vi "Conv2D(LabVIEW).vi"() -> ()   [LabVIEW 2020]
uses:
  725156de-cf75-4898-947e-c29841973b14.vi
  dd0536cf-4951-4d31-99bd-6811dd0ed3e3.vi
  <vilib>/Utility/High Resolution Relative Seconds.vi
  <vilib>/Analysis/baseanly.llb/Mean (DBL).vi
  <vilib>/Analysis/2dsp.llb/2D Convolution (DBL).vi
  <vilib>/Utility/file.llb/Write Delimited Spreadsheet (DBL).vi
  <vilib>/Analysis/NI_AALBase.lvlib
  <vilib>/Analysis/NI_AALPro.lvlib
panel:
  out "Results(s)":dbl[][](array[numeric])=[[0.00042240900000251714, 0.0006797469999992245, 0.001307318000003761, 0.0018059579999999188, 0.0029984490000015285, 0.0035659910000003948, 0.005167819000002964], [0.0016064430000005813, 0.002645904999999402, 0.0053270980000024795, 0.007167966000001798, 0.011575462000000697, 0.01364413499999955, 0.01941537100000005], [0.006691304000000855, 0.010726035000002411, 0.020936882000000878, 0.027458231000000523, 0.04479016899999806, 0.05343978200000038, 0.07617650899999717], [0.027480451999999787, 0.042863392000003844, 0.08360431799999787, 0.11047097800000301, 0.17862831899999945, 0.21162874799999826, 0.29438628300000347], [0.11078803599999901, 0.17429765300000327, 0.331365909000001, 0.4447229849999985, 0.7105940409999993, 0.886198787000003, 1.1901550199999975]] format="%.2f"
  in  "algorithm":enum32{"direct", "frequency domain"}(ring)
  in  "Kernel Size":i32[](array[numeric])=[3, 5, 7, 9, 11, 13, 15]
  in  "Image Size":i32[](array[numeric])=[128, 256, 512, 1024, 2048]
  in  "Batch":i32=100
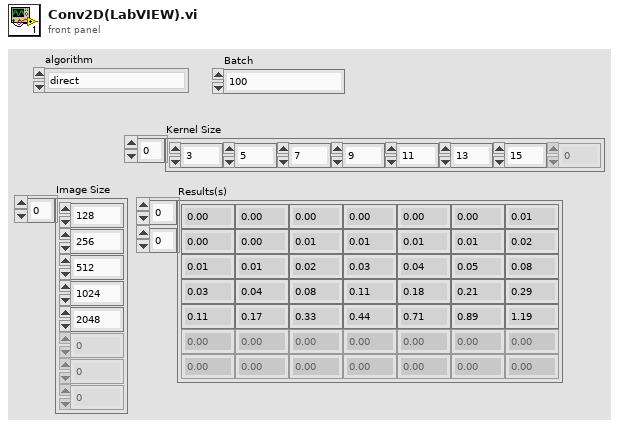
[diagram p1: front panel]
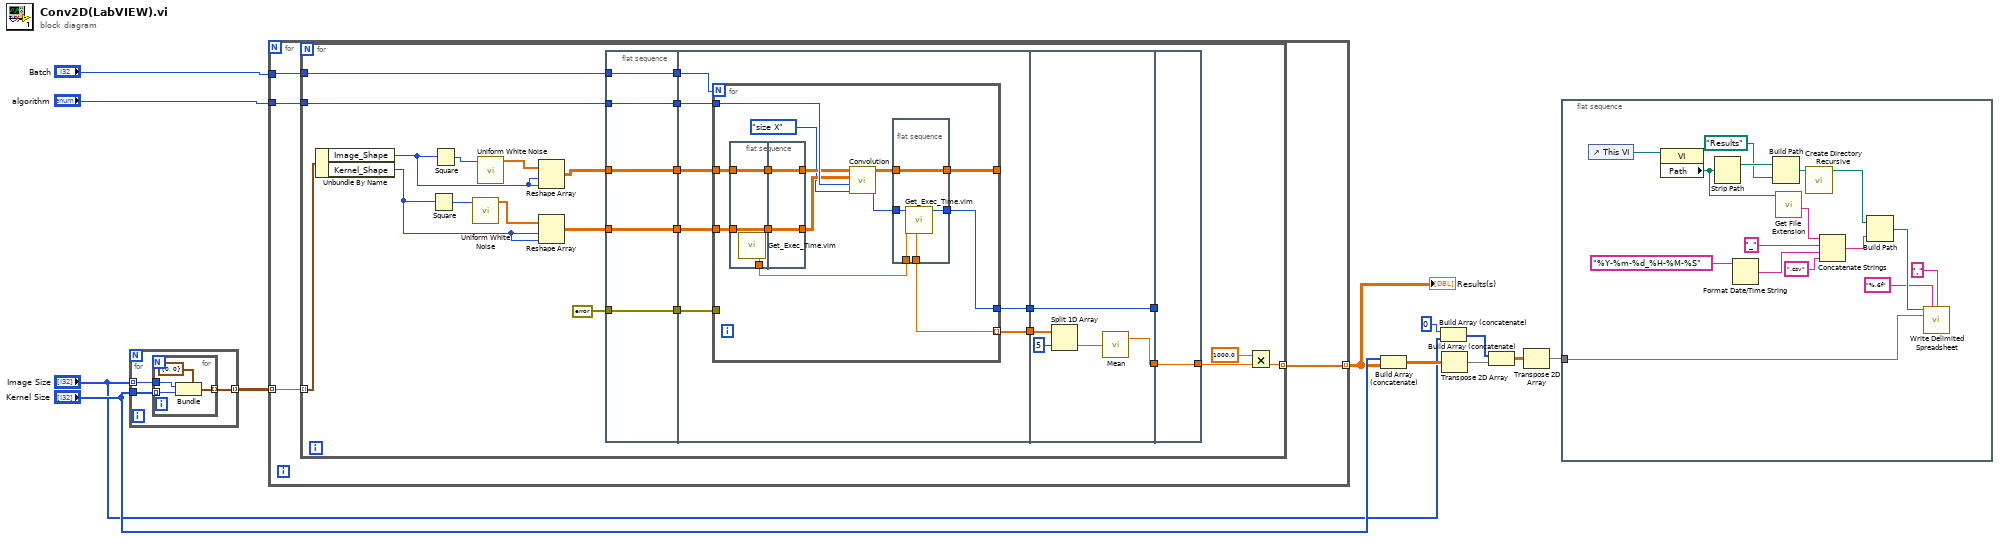
[diagram p0: block diagram]
diagram:
  n1 = for {
    tunnel: "Image Size" -> [w14] mode=indexing
    tunnel: "Kernel Size" -> [w15]
    tunnel: [w13] -> w1 mode=indexing
    n2 = for {
      tunnel: w15 -> [w18] mode=indexing
      tunnel: w14 -> [w19]
      tunnel: [w17] -> w13 mode=indexing
      n3 = Bundle(cluster=cluster{"Image_Shape":i32, "Kernel_Shape":i32} {"Image_Shape"=0, "Kernel_Shape"=0}, "Image_Shape"=w19, "Kernel_Shape"=w18) -> (w17:cluster{"Image_Shape":i32, "Kernel_Shape":i32})
    }
  }
  n4 = for {
    tunnel: w1 -> [w23] mode=indexing
    tunnel: "Batch" -> [w20]
    tunnel: [w22] -> w4 mode=indexing
    tunnel: "algorithm" -> [w21]
    n5 = for {
      tunnel: w23 -> [w47] mode=indexing
      tunnel: [w26] -> w22 mode=indexing
      tunnel: w21 -> [w29]
      tunnel: w20 -> [w28]
      n6 = Unbundle By Name(w47) -> ("Image_Shape"=w38:i32, "Kernel_Shape"=w42:i32)
      n7 = Square(x=w42) -> (x^2=w39:i32)
      n8 = Square(x=w38) -> (x^2=w27:i32)
      n9 = call <vilib>:"Uniform White Noise.vi"("samples"=w39) -> ("uniform white noise"=w40:dbl[])  [unwired: 9 in, 1 out]
      n10 = call <vilib>:"Uniform White Noise.vi"("samples"=w27) -> ("uniform white noise"=w41:dbl[])  [unwired: 9 in, 1 out]
      n11 = Reshape Array(w41, w38, w38) -> (w33:dbl[][])
      n12 = Reshape Array(w40, w42, w42) -> (w43:dbl[][])
      n13 = flat-sequence {
        tunnel: w29 -> [w50]
        tunnel: errorcluster {"status"=FALSE, "code"=0, "source"=""} ("error out") -> [w49]
        tunnel: w43 -> [w51]
        tunnel: w33 -> [w52]
        tunnel: [w52] -> w37
        tunnel: [w51] -> w36
        tunnel: [w49] -> w35
        tunnel: [w50] -> w34
        tunnel: [w48] -> w32
        tunnel: w28 -> [w48]
        tunnel: [w56] -> w46
        tunnel: w37 -> [w59]
        tunnel: w36 -> [w58]
        tunnel: w35 -> [w57]
        tunnel: w34 -> [w55]
        tunnel: w32 -> [w54]
        tunnel: [w53] -> w31
        tunnel: w46 -> [w88]
        tunnel: [w88] -> w44
        tunnel: w31 -> [w87]
        tunnel: [w84] -> w30
        tunnel: [w89] -> w45
        tunnel: w44 -> [_]
        tunnel: w30 -> [w89]
        frame #0 {
        }
        frame #1 {
          n14 = for {
            N: w54 -> [_]
            tunnel: w59 -> [w66]
            tunnel: w58 -> [w67]
            tunnel: w57 -> [_]
            tunnel: [w73] -> w56
            tunnel: w55 -> [w71]
            tunnel: [w70] -> _
            tunnel: [w68] -> w53 mode=indexing
            n15 = flat-sequence {
              tunnel: w66 -> [w75]
              tunnel: w67 -> [w76]
              tunnel: [w76] -> w63
              tunnel: [w75] -> w62
              tunnel: [w74] -> w61
              tunnel: [w77] -> w65
              tunnel: [w78] -> w64
              tunnel: w63 -> [w77]
              tunnel: w62 -> [w78]
              frame #0 {
                n16 = call "Get_Exec_Time.vim"() -> ("T(n)"=w74:dbl)  [unwired: 7 in, 2 out]
              }
              frame #1 {
              }
            }
            n17 = call-poly <vilib>:"Convolution.vi"("output size"=enum32{"full", "size X", "compact"}."size X", "algorithm"=w71, "Y"=w65, "X"=w64) -> ("error"=w72:i32, "X * Y"=w69:dbl[][])  [unwired: 6 in]
            n18 = flat-sequence {
              tunnel: [w82] -> w70
              tunnel: [w81] -> w73
              tunnel: w61 -> [w80]
              tunnel: [w79] -> w68
              tunnel: w72 -> [w83]
              tunnel: w69 -> [w82]
              frame #0 {
                n19 = call "Get_Exec_Time.vim"("T(n-1)"=w80, "error in (no error)"=w83) -> ("error out"=w81:i32, "dT"=w79:dbl)  [unwired: 5 in, 1 out]
              }
            }
          }
        }
        frame #2 {
          n20 = Split 1D Array(array=w87, index=5) -> (second subarray=w85:dbl[])  [unwired: 1 out]
          n21 = call-poly <vilib>:"Mean.vi"("X"=w85) -> ("mean"=w84:dbl)  [unwired: 1 out]
        }
        frame #3 {
        }
      }
      n22 = Multiply(x=1000.0, y=w45) -> (x*y=w26:dbl)
    }
  }
  "Results(s)" <- w4
  n23 = Build Array (concatenate)("Kernel Size", w4) -> (w12:dbl[][])
  n24 = Build Array (concatenate)(0 ("element"), "Image Size") -> (w8:i32[])
  n25 = Transpose 2D Array(2D array=w12) -> (transposed array=w10:dbl[][])
  n26 = Build Array (concatenate)(w8, w10) -> (w9:dbl[][])
  n27 = Transpose 2D Array(2D array=w9) -> (transposed array=w5:dbl[][])
  n28 = flat-sequence {
    tunnel: w5 -> [w105]
    frame #0 {
      n29 = control-ref of="This VI"() -> (w98:refnum<vi>)
      n30 = property class="VI"(reference=w98) -> ("Path"=w93:path)  [unwired: 1 in, 2 out]
      n31 = Strip Path(path=w93) -> (stripped path=w97:path)  [unwired: 1 out]
      n32 = Format Date/Time String(time format string (%c)="%Y-%m-%d_%H-%M-%S") -> (date/time string=w100:string)  [unwired: 2 in]
      n33 = Build Path(base path=w97, name or relative path=path "Results") -> (appended path=w96:path)
      n34 = call <vilib>:"Get File Extension.vi"("file"=w93) -> ("filename without extension"=w92:string)  [unwired: 6 in, 4 out]
      n35 = call <vilib>:"Create Directory Recursive.vi"("directory"=w96) -> ("directory copy"=w94:path)  [unwired: 4 in, 2 out]
      n36 = Concatenate Strings(w92, "_" ("string"), w100, ".csv" ("string")) -> (w102:string)
      n37 = Build Path(base path=w94, name or relative path=w102) -> (appended path=w103:path)
      n38 = call-poly <vilib>:"Write Delimited Spreadsheet.vi"("file path (dialog if empty)"=w103, "format (%.3f)"="%.6f", "2D data"=w105, "delimiter (\\t)"="," ("delimiter (\\t)")) -> ()  [unwired: 10 in, 2 out]
    }
  }
